vi "TempRamp.vi"(0 "IP Address":string="192.168.12.200", 1 "Temperature Log Interval (s)":dbl=10.0, 2 "Path to Temp Log Folder":string="C:\\Users\\ErNa\\Documents\\LabView Codes\\ErNa Sodium Oven Controller\\Temperature Logs\\Ramp_", 5 "Port Number":u16=2000, 7 "Start Temperature (C)":dbl, 9 "End Temperature (C)":dbl=9.0, 11 "Duration of Ramp (min)":dbl=5.0, 12 "Error In (no error)":errorcluster) -> (4 "Current Temperature (C)":dbl=8.0 format="%.2f", 6 "Setpoint Diagnosis":string="W01\r\n", 8 "Temp Log Diagnosis":path=path "C:/Users/ErNa/Documents/LabView Codes/ErNa Sodium Oven Controller/Temperature Logs/Ramp_Tue, Feb 12, 2019_12-50 PM.xlsx" caption="Filename Out", 14 "Error Out":errorcluster)   [LabVIEW 2013, in "ovenCtrl.lvlib"]
uses:
  ovenCtrl.lvlib
panel:
  # "Inputs"
  # "Device Address"
  # "Temperature Ramp"
  # "Outputs"
  # "Diagnosis"
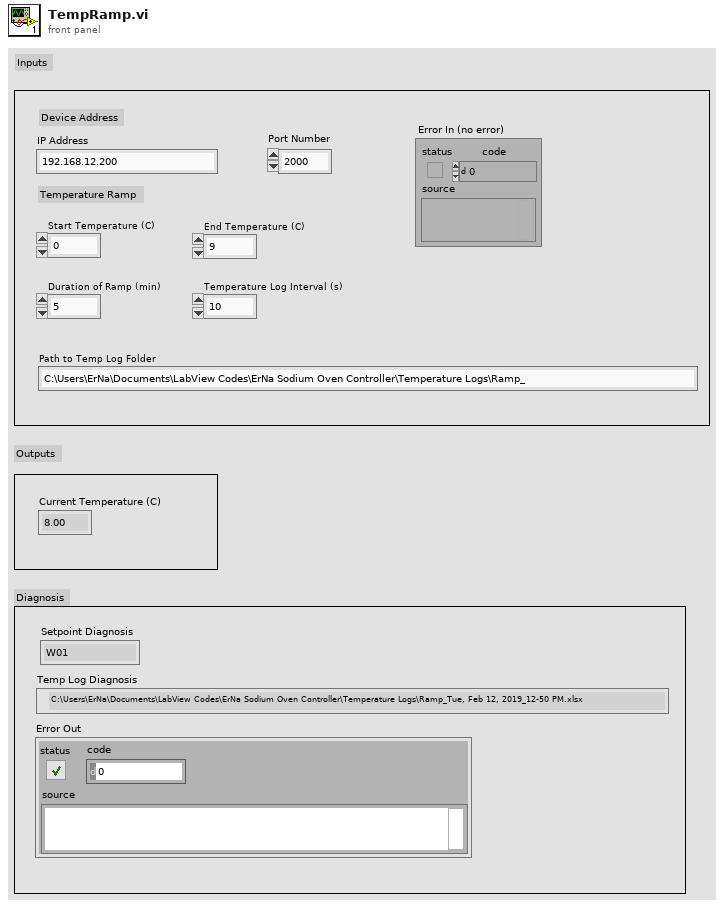
[diagram p1: front panel]
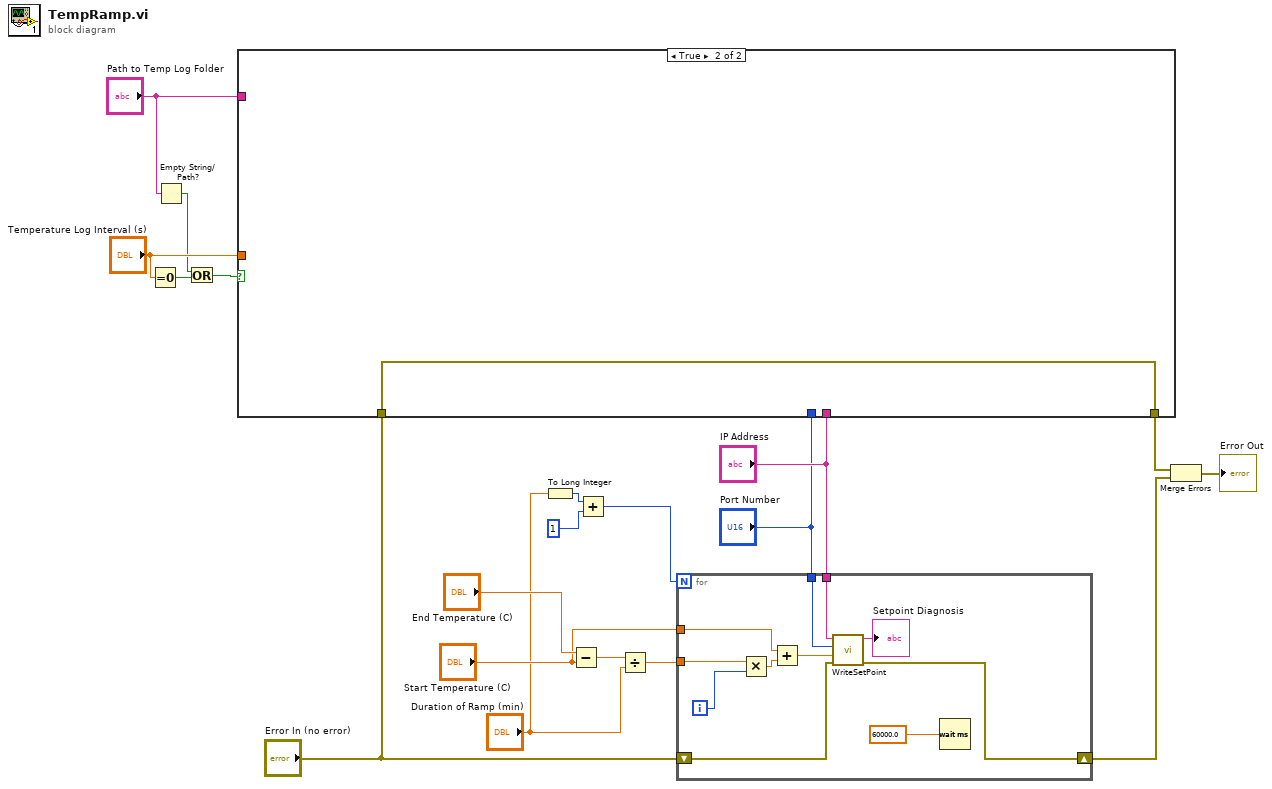
[diagram p0: block diagram]
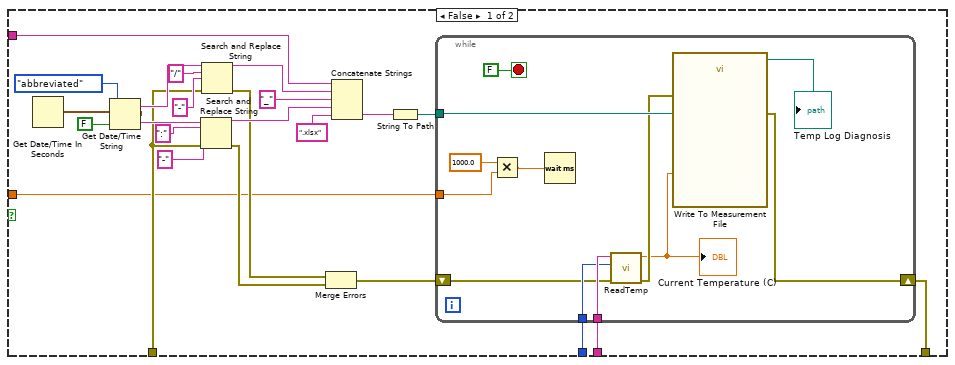
[diagram p2: hidden frame]
diagram:
  n1 = Equal To 0?(x="Temperature Log Interval (s)") -> (x = 0?=w3:bool)
  n2 = Empty String/Path?(string/path="Path to Temp Log Folder") -> (empty?=w2:bool)
  n3 = Or(x=w2, y=w3) -> (x .or. y?=w1:bool)
  n4 = case shown="True" w1 {
    tunnel: "IP Address" -> [w43 _]
    tunnel: "Port Number" -> [w42 _]
    tunnel: "Error In (no error)" -> [w28 w56]
    tunnel: [w22 w56] -> w8
    tunnel: "Path to Temp Log Folder" -> [w21 _]
    tunnel: "Temperature Log Interval (s)" -> [w20 _]
    frame False {
      n5 = Get Date/Time In Seconds() -> (seconds since 1Jan1904=w26:timestamp)
      n6 = Get Date/Time String(date format (0)=enum16{"short", "long", "abbreviated"}."abbreviated", seconds (now)=w26, want seconds? (F)=FALSE) -> (date string=w37:string, time string=w32:string)
      n7 = Search and Replace String(input string=w32, search string=":", replace string="-" ("replace string (\"\")"), error in=w28) -> (result string=w29:string, error out=w24:errorcluster)  [unwired: 4 in, 2 out]
      n8 = Search and Replace String(input string=w37, search string="/", replace string="-" ("replace string (\"\")"), error in=w28) -> (result string=w34:string, error out=w25:errorcluster)  [unwired: 4 in, 2 out]
      n9 = Merge Errors(w25, w24) -> (w23:errorcluster)
      n10 = Concatenate Strings(w21, w34, "_" ("string"), w29, ".xlsx" ("string")) -> (w40:string)
      n11 = String To Path(string=w40) -> (path=w39:path)
      n12 = while {
        tunnel: w20 -> [w52]
        tunnel: w43 -> [w54]
        tunnel: w42 -> [w53]
        tunnel: w39 -> [w50]
        shift-right: [w47] -> w22
        shift-left: w23 -> [w48]
        stop <- FALSE stop-if-true
        n13 = Multiply(x=1000.0 ("y"), y=w52) -> (x*y=w55:dbl)
        n14 = Wait (ms)(milliseconds to wait=w55) -> ()  [unwired: 1 out]
        n15 = call "ReadTemp.vi"("error in (no error)"=w48, "Port Number"=w53, "IP Address"=w54) -> ("error out"=w49:errorcluster, "Temperature"=w45:dbl)  [unwired: 7 in]
        "Current Temperature (C)" <- w45
        n16 = call "Write To Measurement File"("Signals"=w45, "error in (no error)"=w49, "Filename"=w50) -> ("Filename Out"=→"Temp Log Diagnosis":path, "error out"=w47:errorcluster)  [unwired: 14 in, 1 out]
      }
    }
    frame True {
    }
  }
  n17 = To Long Integer(number="Duration of Ramp (min)") -> (32bit integer=w14:i32)
  n18 = Subtract(x="End Temperature (C)", y="Start Temperature (C)") -> (x-y=w18:dbl)
  n19 = Add(x=w14, y=1) -> (x+y=w12:i32)
  n20 = Divide(x=w18, y="Duration of Ramp (min)") -> (x/y=w16:dbl)
  n21 = for {
    N: w12 -> [_]
    tunnel: "Start Temperature (C)" -> [w67]
    tunnel: w16 -> [w61]
    tunnel: "IP Address" -> [w63]
    tunnel: "Port Number" -> [w62]
    shift-right: [w58] -> w7
    shift-left: "Error In (no error)" -> [w59]
    i -> [w66]
    n22 = Multiply(x=w61, y=w66) -> (x*y=w65:dbl)
    n23 = Add(x=w67, y=w65) -> (x+y=w64:dbl)
    n24 = call "WriteSetPoint.vi"("error in (no error)"=w59, "Setpoint (C)"=w64, "Port Number"=w62, "IP Address"=w63) -> ("error out"=w58:errorcluster, "Output Reading"=→"Setpoint Diagnosis":string)  [unwired: 6 in]
    n25 = Wait (ms)(milliseconds to wait=60000.0 ("y")) -> ()  [unwired: 1 out]
  }
  n26 = Merge Errors(w8, w7) -> (→"Error Out":errorcluster)
